vi "UiSchematic_gm.vi"() -> ()   [LabVIEW 2011]
uses:
  Pumpe.ctl
  Output - Cluster gas.ctl
panel:
  out "status":string
  out "Raumtemperatur \nTS-2 [°C]":dbl format="%.2g"
  out "B2G1 HR V1":bool
  out "Fab2 MR V1":bool
  out "B2G1 MR V1":bool
  out "B2G2 T2 V1":bool
  out "B2G2 MR V1":bool
  out "B2G1 T2 V1":bool
  out "Fab1 BL V1":bool
  out "Fab1 HR V1":bool
  out "Fab1 MR V1":bool
  out "Fab2 HR V1":bool
  out "DS-2 [bar]":dbl format="%.4g"
  out "GZ-1 [l]":dbl format="%.2f"
  out "DS-1 [bar]":dbl format="%.4g"
  out "TS-1 [°C]":dbl format="%.2g"
  out "cRio":timestamp
  out "GM P-2":bool
  out "PC":timestamp
  out "GM V-1":bool
  out "GM V-4":bool
  out "GM V-3":bool
  out "GM V-2":bool
  out "h2 [%]":dbl format="%.2g"
  out "co2 [%]":dbl format="%.2g"
  out "ch4 [%]":dbl format="%.2g"
  out "GM P-1":T1
  out "B2G1 HR V1.1":bool
  out "Fab2 MR V1.1":bool
  out "B2G1 MR V1.1":bool
  out "B2G2 T2 V1.1":bool
  out "B2G2 MR V1.1":bool
  out "B2G1 T2 V1.1":bool
  out "Fab1 BL V1.1":bool
  out "Fab1 HR V1.1":bool
  out "Fab1 MR V1.1":bool
  out "Fab2 HR V1.1":bool
  in  "stop":bool
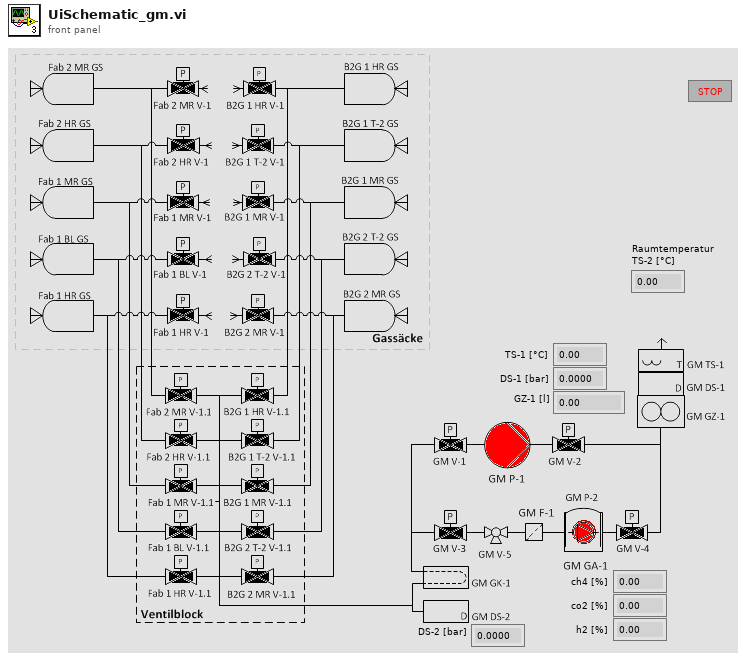
[diagram p1: front panel]
types:
  T1 = typedef "Pumpe.ctl" = bool
  T2 = typedef "Output - Cluster gas.ctl" = cluster{"B2G2 MR V1.1 AUF":bool, "B2G2 MR V1.1 ZU":bool, "B2G2 MR V1 AUF":bool, "B2G2 MR V1 ZU":bool, "B2G1 T2 V1 AUF":bool, "B2G1 T2 V1 ZU":bool, "B2G1 T2 V1.1 AUF":bool, "B2G1 T2 V1.1 ZU":bool, "B2G2 T2 V1 AUF":bool, "B2G2 T2 V1 ZU":bool, "B2G2 T2 V1.1 ZU":bool, "B2G2 T2 V1.1 AUF":bool, "B2G1 MR V1 AUF":bool, "B2G1 MR V1 ZU":bool, "B2G1 MR V1.1 AUF":bool, "B2G1 MR V1.1 ZU":bool, "B2G1 HR V1 AUF":bool, "B2G1 HR V1 ZU":bool, "B2G1 HR V1.1 AUF":bool, "B2G1 HR V1.1 ZU":bool, "Fab1 HR V1 AUF":bool, "Fab1 HR V1 ZU":bool, "Fab1 HR V1.1 AUF":bool, "Fab1 HR V1.1 ZU":bool, "Fab1 MR V1 AUF":bool, "Fab1 MR V1 ZU":bool, "Fab1 MR V1.1 AUF":bool, "Fab1 MR V1.1 ZU":bool, "Fab1 BL V1 AUF":bool, "Fab1 BL V1 ZU":bool, "Fab1 BL V1.1 AUF":bool, "Fab1 BL V1.1 ZU":bool, "Fab2 HR V1 AUF":bool, "Fab2 HR V1 ZU":bool, "Fab2 HR V1.1 AUF":bool, "Fab2 HR V1.1 ZU":bool, "Fab2 MR V1 AUF":bool, "Fab2 MR V1 ZU":bool, "Fab2 MR V1.1 AUF":bool, "Fab2 MR V1.1 ZU":bool, "GA1 ch4 [%]":dbl, "GA1 co2 [%]":dbl, "GA1 h2 [%]":dbl, "GM P1 RUN":bool, "GM V-1 AUF":bool, "GM V-1 ZU":bool, "GM V-2 AUF":bool, "GM V-2 ZU":bool, "GM V-3 AUF":bool, "GM V-3 ZU":bool, "GM V-4 AUF":bool, "GM V-4 ZU":bool, "GM P2 RUN":bool, "GM GZ-1 [imp]":u32, "GM DS-2 [bar]":dbl, "GM DS-1 [bar]":dbl, "GM TS-1 [°C]":dbl, "GM TS-2[°C]":dbl, "gas_values":cluster{"timestamp":timestamp, "GM DS-2 [bar]":dbl, "GA1 ch4 [%]":dbl, "GA1 co2 [%]":dbl, "GA1 h2 [%]":dbl, "GM DS-1 [bar]":dbl, "GM TS-1 [°C]":dbl, "GM TS-2 [°C]":dbl, "GM GZ-1 [l]":dbl, "empty":bool, "measuring point":u8}, "measuring mode":u8}
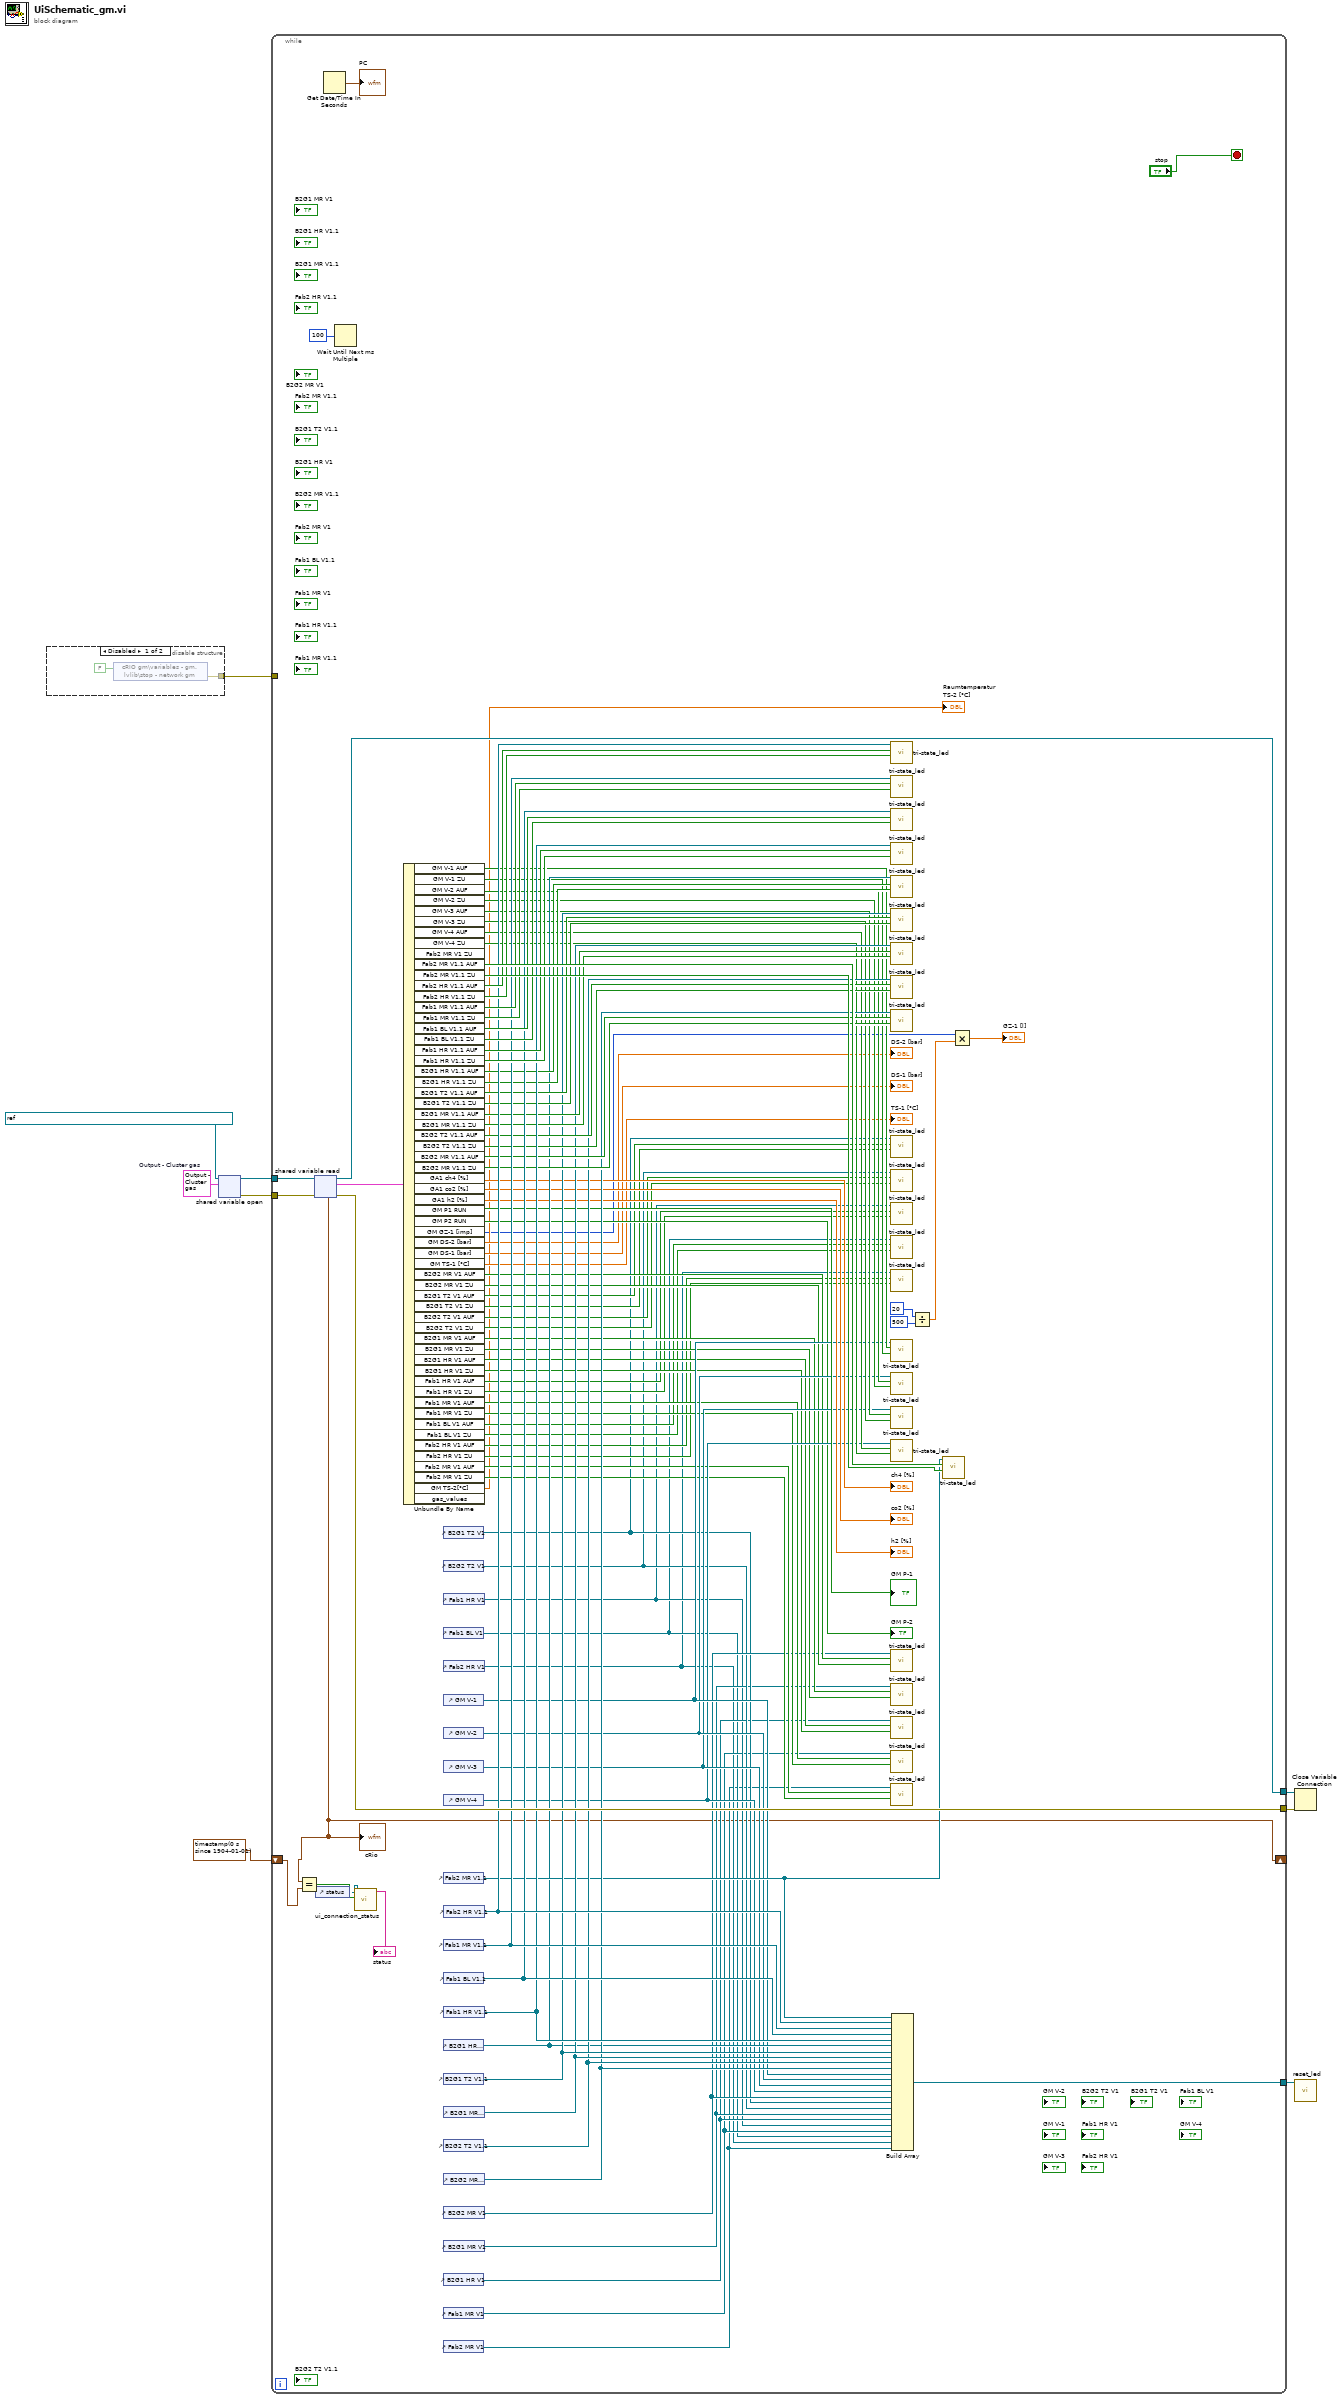
[diagram p0: block diagram]
diagram:
  w6 = T2 {"B2G2 MR V1.1 AUF"=FALSE, "B2G2 MR V1.1 ZU"=FALSE, "B2G2 MR V1 AUF"=FALSE, "B2G2 MR V1 ZU"=FALSE, "B2G1 T2 V1 AUF"=FALSE, "B2G1 T2 V1 ZU"=FALSE, "B2G1 T2 V1.1 AUF"=FALSE, "B2G1 T2 V1.1 ZU"=FALSE, "B2G2 T2 V1 AUF"=FALSE, "B2G2 T2 V1 ZU"=FALSE, "B2G2 T2 V1.1 ZU"=FALSE, "B2G2 T2 V1.1 AUF"=FALSE, "B2G1 MR V1 AUF"=FALSE, "B2G1 MR V1 ZU"=FALSE, "B2G1 MR V1.1 AUF"=FALSE, "B2G1 MR V1.1 ZU"=FALSE, "B2G1 HR V1 AUF"=FALSE, "B2G1 HR V1 ZU"=FALSE, "B2G1 HR V1.1 AUF"=FALSE, "B2G1 HR V1.1 ZU"=FALSE, "Fab1 HR V1 AUF"=FALSE, "Fab1 HR V1 ZU"=FALSE, "Fab1 HR V1.1 AUF"=FALSE, "Fab1 HR V1.1 ZU"=FALSE, "Fab1 MR V1 AUF"=FALSE, "Fab1 MR V1 ZU"=FALSE, "Fab1 MR V1.1 AUF"=FALSE, "Fab1 MR V1.1 ZU"=FALSE, "Fab1 BL V1 AUF"=FALSE, "Fab1 BL V1 ZU"=FALSE, "Fab1 BL V1.1 AUF"=FALSE, "Fab1 BL V1.1 ZU"=FALSE, "Fab2 HR V1 AUF"=FALSE, "Fab2 HR V1 ZU"=FALSE, "Fab2 HR V1.1 AUF"=FALSE, "Fab2 HR V1.1 ZU"=FALSE, "Fab2 MR V1 AUF"=FALSE, "Fab2 MR V1 ZU"=FALSE, "Fab2 MR V1.1 AUF"=FALSE, "Fab2 MR V1.1 ZU"=FALSE, "GA1 ch4 [%]"=0.0, "GA1 co2 [%]"=0.0, "GA1 h2 [%]"=0.0, "GM P1 RUN"=FALSE, "GM V-1 AUF"=FALSE, "GM V-1 ZU"=FALSE, "GM V-2 AUF"=FALSE, "GM V-2 ZU"=FALSE, "GM V-3 AUF"=FALSE, "GM V-3 ZU"=FALSE, "GM V-4 AUF"=FALSE, "GM V-4 ZU"=FALSE, "GM P2 RUN"=FALSE, "GM GZ-1 [imp]"=0, "GM DS-2 [bar]"=0.0, "GM DS-1 [bar]"=0.0, "GM TS-1 [°C]"=0.0, "GM TS-2[°C]"=0.0, "gas_values"={"timestamp"=timestamp(0 s since 1904-01-01), "GM DS-2 [bar]"=0.0, "GA1 ch4 [%]"=0.0, "GA1 co2 [%]"=0.0, "GA1 h2 [%]"=0.0, "GM DS-1 [bar]"=0.0, "GM TS-1 [°C]"=0.0, "GM TS-2 [°C]"=0.0, "GM GZ-1 [l]"=0.0, "empty"=FALSE, "measuring point"=0}, "measuring mode"=0}  # Output - Cluster gas
  n1 = disable-structure shown="Disabled" {
    disable-tunnel: [w11 _] -> w2
    frame Disabled {
      n2 = shared-variable "cRIO gm\\variables - gm.lvlib\\stop - network gm"(FALSE ("stop - network gas")) -> (error out=w11:errorcluster)  [unwired: 1 in]
    }
    frame Enabled {
    }
  }
  n3 = shared-variable-open(refnum<k21> "ni.var.psp://10.27.40.21/variables - gm/data - network - gm" ("Output Var gas"), w6) -> (w4:refnum<k21>, w3:errorcluster)  [unwired: 2 in]
  n4 = while {
    tunnel: w4 -> [w111]
    tunnel: [w110] -> w8
    tunnel: w3 -> [w108]
    tunnel: [w107] -> w7
    tunnel: [w91] -> w5
    tunnel: w2 -> [_]
    shift-right: [w14] -> _
    shift-left: timestamp(0 s since 1904-01-01) -> [w15]
    stop <- "stop" stop-if-true
    n5 = shared-variable-read(w111, w108) -> (w110:refnum<k21>, w107:errorcluster, w109:T2, w14:timestamp)
    "cRio" <- w14
    n6 = Equal?(x=w14, y=w15) -> (x = y?=w16:bool)
    n7 = control-ref of="status"() -> (w13:refnum<vi>)
    n8 = Get Date/Time In Seconds() -> (seconds since 1Jan1904=→"PC":timestamp)
    n9 = Wait Until Next ms Multiple(millisecond multiple=u32 100) -> ()  [unwired: 1 out]
    n10 = call "ui_connection_status.vi"("Boolean"=w16, "String in"=w13) -> ("status"=→"status":string)  [unwired: 9 in]
    n11 = Unbundle By Name(w109) -> ("GM V-1 AUF"=w70:bool, "GM V-1 ZU"=w69:bool, "GM V-2 AUF"=w68:bool, "GM V-2 ZU"=w67:bool, "GM V-3 AUF"=w66:bool, "GM V-3 ZU"=w65:bool, "GM V-4 AUF"=w64:bool, "GM V-4 ZU"=w63:bool, "Fab2 MR V1.1 AUF"=w105:bool, "Fab2 MR V1.1 ZU"=w104:bool, "Fab2 HR V1.1 AUF"=w103:bool, "Fab2 HR V1.1 ZU"=w102:bool, "Fab1 MR V1.1 AUF"=w101:bool, "Fab1 MR V1.1 ZU"=w100:bool, "Fab1 BL V1.1 AUF"=w99:bool, "Fab1 BL V1.1 ZU"=w98:bool, "Fab1 HR V1.1 AUF"=w97:bool, "Fab1 HR V1.1 ZU"=w96:bool, "B2G1 HR V1.1 AUF"=w90:bool, "B2G1 HR V1.1 ZU"=w89:bool, "B2G1 T2 V1.1 AUF"=w88:bool, "B2G1 T2 V1.1 ZU"=w87:bool, "B2G1 MR V1.1 AUF"=w86:bool, "B2G1 MR V1.1 ZU"=w85:bool, "B2G2 T2 V1.1 AUF"=w84:bool, "B2G2 T2 V1.1 ZU"=w83:bool, "B2G2 MR V1.1 AUF"=w82:bool, "B2G2 MR V1.1 ZU"=w81:bool, "GA1 ch4 [%]"=→"ch4 [%]":dbl, "GA1 co2 [%]"=→"co2 [%]":dbl, "GA1 h2 [%]"=→"h2 [%]":dbl, "GM P1 RUN"=→"GM P-1":bool, "GM P2 RUN"=→"GM P-2":bool, "GM GZ-1 [imp]"=w21:u32, "GM DS-2 [bar]"=→"DS-2 [bar]":dbl, "GM DS-1 [bar]"=→"DS-1 [bar]":dbl, "GM TS-1 [°C]"=→"TS-1 [°C]":dbl, "B2G2 MR V1 AUF"=w53:bool, "B2G2 MR V1 ZU"=w52:bool, "B2G1 T2 V1 AUF"=w51:bool, "B2G1 T2 V1 ZU"=w50:bool, "B2G2 T2 V1 AUF"=w49:bool, "B2G2 T2 V1 ZU"=w48:bool, "B2G1 MR V1 AUF"=w47:bool, "B2G1 MR V1 ZU"=w46:bool, "B2G1 HR V1 AUF"=w45:bool, "B2G1 HR V1 ZU"=w44:bool, "Fab1 HR V1 AUF"=w43:bool, "Fab1 HR V1 ZU"=w42:bool, "Fab1 MR V1 AUF"=w41:bool, "Fab1 MR V1 ZU"=w40:bool, "Fab1 BL V1 AUF"=w39:bool, "Fab1 BL V1 ZU"=w38:bool, "Fab2 HR V1 AUF"=w37:bool, "Fab2 HR V1 ZU"=w36:bool, "Fab2 MR V1 AUF"=w35:bool, "Fab2 MR V1 ZU"=w34:bool, "GM TS-2[°C]"=→"Raumtemperatur \nTS-2 [°C]":dbl)  [unwired: 2 out]
    n12 = control-ref of="B2G1 T2 V1"() -> (w32:refnum<vi>)
    n13 = control-ref of="B2G2 T2 V1"() -> (w31:refnum<vi>)
    n14 = control-ref of="Fab1 BL V1"() -> (w26:refnum<vi>)
    n15 = control-ref of="GM V-1"() -> (w62:refnum<vi>)
    n16 = control-ref of="GM V-2"() -> (w61:refnum<vi>)
    n17 = control-ref of="GM V-3"() -> (w60:refnum<vi>)
    n18 = control-ref of="GM V-4"() -> (w59:refnum<vi>)
    n19 = control-ref of="Fab2 MR V1.1"() -> (w76:refnum<vi>)
    n20 = control-ref of="Fab1 MR V1.1"() -> (w94:refnum<vi>)
    n21 = control-ref of="Fab1 BL V1.1"() -> (w93:refnum<vi>)
    n22 = control-ref of="B2G1 HR V1.1"() -> (w75:refnum<vi>)
    n23 = control-ref of="B2G1 T2 V1.1"() -> (w80:refnum<vi>)
    n24 = control-ref of="B2G2 T2 V1.1"() -> (w78:refnum<vi>)
    n25 = control-ref of="B2G1 HR V1"() -> (w29:refnum<vi>)
    n26 = control-ref of="Fab1 MR V1"() -> (w27:refnum<vi>)
    n27 = control-ref of="Fab2 MR V1"() -> (w24:refnum<vi>)
    n28 = control-ref of="Fab1 HR V1"() -> (w28:refnum<vi>)
    n29 = control-ref of="Fab2 HR V1"() -> (w25:refnum<vi>)
    n30 = control-ref of="Fab2 HR V1.1"() -> (w95:refnum<vi>)
    n31 = control-ref of="Fab1 HR V1.1"() -> (w92:refnum<vi>)
    n32 = control-ref of="B2G1 MR V1.1"() -> (w79:refnum<vi>)
    n33 = control-ref of="B2G2 MR V1.1"() -> (w77:refnum<vi>)
    n34 = control-ref of="B2G2 MR V1"() -> (w33:refnum<vi>)
    n35 = control-ref of="B2G1 MR V1"() -> (w30:refnum<vi>)
    n36 = call "tri-state_led.vi"("CLOSE"=w102, "OPEN"=w103, "ref in"=w95) -> ()  [unwired: 9 in]
    n37 = call "tri-state_led.vi"("CLOSE"=w100, "OPEN"=w101, "ref in"=w94) -> ()  [unwired: 9 in]
    n38 = call "tri-state_led.vi"("CLOSE"=w98, "OPEN"=w99, "ref in"=w93) -> ()  [unwired: 9 in]
    n39 = call "tri-state_led.vi"("CLOSE"=w96, "OPEN"=w97, "ref in"=w92) -> ()  [unwired: 9 in]
    n40 = call "tri-state_led.vi"("CLOSE"=w89, "OPEN"=w90, "ref in"=w75) -> ()  [unwired: 9 in]
    n41 = call "tri-state_led.vi"("CLOSE"=w87, "OPEN"=w88, "ref in"=w80) -> ()  [unwired: 9 in]
    n42 = call "tri-state_led.vi"("CLOSE"=w85, "OPEN"=w86, "ref in"=w79) -> ()  [unwired: 9 in]
    n43 = call "tri-state_led.vi"("CLOSE"=w83, "OPEN"=w84, "ref in"=w78) -> ()  [unwired: 9 in]
    n44 = call "tri-state_led.vi"("CLOSE"=w81, "OPEN"=w82, "ref in"=w77) -> ()  [unwired: 9 in]
    n45 = call "tri-state_led.vi"("CLOSE"=w50, "OPEN"=w51, "ref in"=w32) -> ()  [unwired: 9 in]
    n46 = call "tri-state_led.vi"("CLOSE"=w48, "OPEN"=w49, "ref in"=w31) -> ()  [unwired: 9 in]
    n47 = call "tri-state_led.vi"("CLOSE"=w42, "OPEN"=w43, "ref in"=w28) -> ()  [unwired: 9 in]
    n48 = call "tri-state_led.vi"("CLOSE"=w38, "OPEN"=w39, "ref in"=w26) -> ()  [unwired: 9 in]
    n49 = call "tri-state_led.vi"("CLOSE"=w36, "OPEN"=w37, "ref in"=w25) -> ()  [unwired: 9 in]
    n50 = call "tri-state_led.vi"("CLOSE"=w69, "OPEN"=w70, "ref in"=w62) -> ()  [unwired: 9 in]
    n51 = call "tri-state_led.vi"("CLOSE"=w67, "OPEN"=w68, "ref in"=w61) -> ()  [unwired: 9 in]
    n52 = call "tri-state_led.vi"("CLOSE"=w65, "OPEN"=w66, "ref in"=w60) -> ()  [unwired: 9 in]
    n53 = call "tri-state_led.vi"("CLOSE"=w63, "OPEN"=w64, "ref in"=w59) -> ()  [unwired: 9 in]
    n54 = call "tri-state_led.vi"("CLOSE"=w52, "OPEN"=w53, "ref in"=w33) -> ()  [unwired: 9 in]
    n55 = call "tri-state_led.vi"("CLOSE"=w46, "OPEN"=w47, "ref in"=w30) -> ()  [unwired: 9 in]
    n56 = call "tri-state_led.vi"("CLOSE"=w44, "OPEN"=w45, "ref in"=w29) -> ()  [unwired: 9 in]
    n57 = call "tri-state_led.vi"("CLOSE"=w40, "OPEN"=w41, "ref in"=w27) -> ()  [unwired: 9 in]
    n58 = call "tri-state_led.vi"("CLOSE"=w34, "OPEN"=w35, "ref in"=w24) -> ()  [unwired: 9 in]
    n59 = Build Array(w76, w95, w94, w93, w92, w75, w80, w79, w78, w77, w62, w61, w60, w59, w33, w32, w31, w30, w29, w28, w27, w26, w25, w24) -> (w91:refnum<vi>[])
    n60 = Divide(x=u32 20, y=u32 500) -> (x/y=w19:dbl)
    n61 = call "tri-state_led.vi"("CLOSE"=w104, "OPEN"=w105, "ref in"=w76) -> ()  [unwired: 9 in]
    n62 = Multiply(x=w21, y=w19) -> (x*y=→"GZ-1 [l]":dbl)
  }
  n63 = Close Variable Connection(8:w7, 11:w8) -> ()  [unwired: 1 out]
  n64 = call "reset_led.vi"("Array"=w5) -> ()  [unwired: 11 in]
